vi "zad1.vi"() -> ()   [LabVIEW 2018]
uses:
  <vilib>/Instr/_visa.llb/VISA Configure Serial Port (Instr).vi
  <vilib>/measure/maspectr.llb/FFT Power Spectrum and PSD for 1 Chan.vi
  <vilib>/measure/NI_MAPro.lvlib
panel:
  out "Waveform Graph":cluster{"f0":dbl, "df":dbl, "magnitude":dbl[]}(graph)
  out "1/x":dbl
  in  "dt":dbl
  out "Waveform Graph 2":dbl[](graph)
  out "Waveform Chart 2":dbl(graph)
  out "Waveform Chart":cluster{dbl, dbl, dbl}(graph)
  in  "stop":bool
  in  "baud rate (9600)":u32=9600
  in  "VISA resource name":refnum<visa-resource-name>
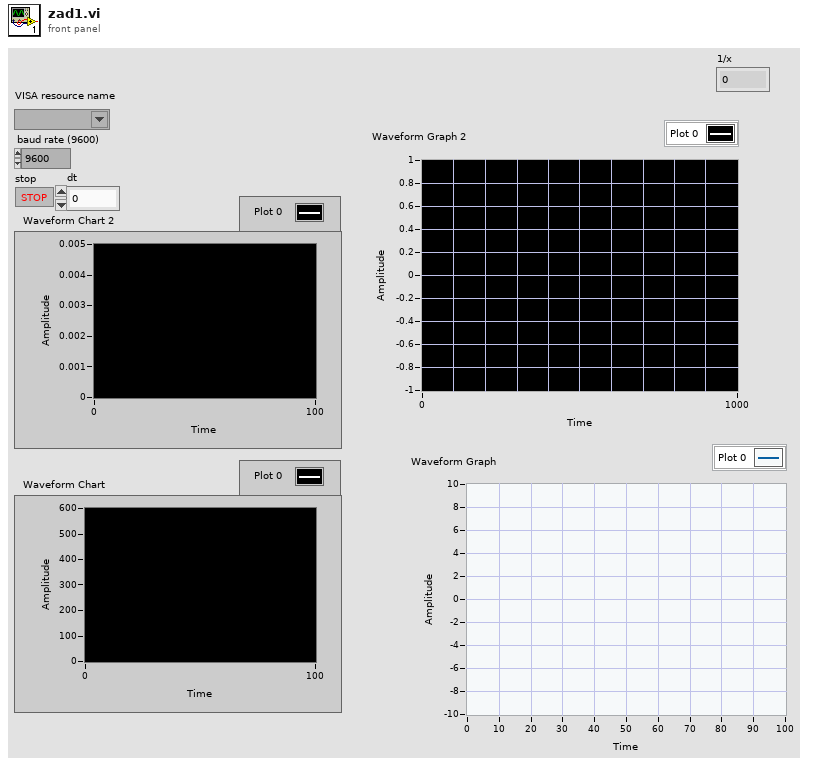
[diagram p1: front panel]
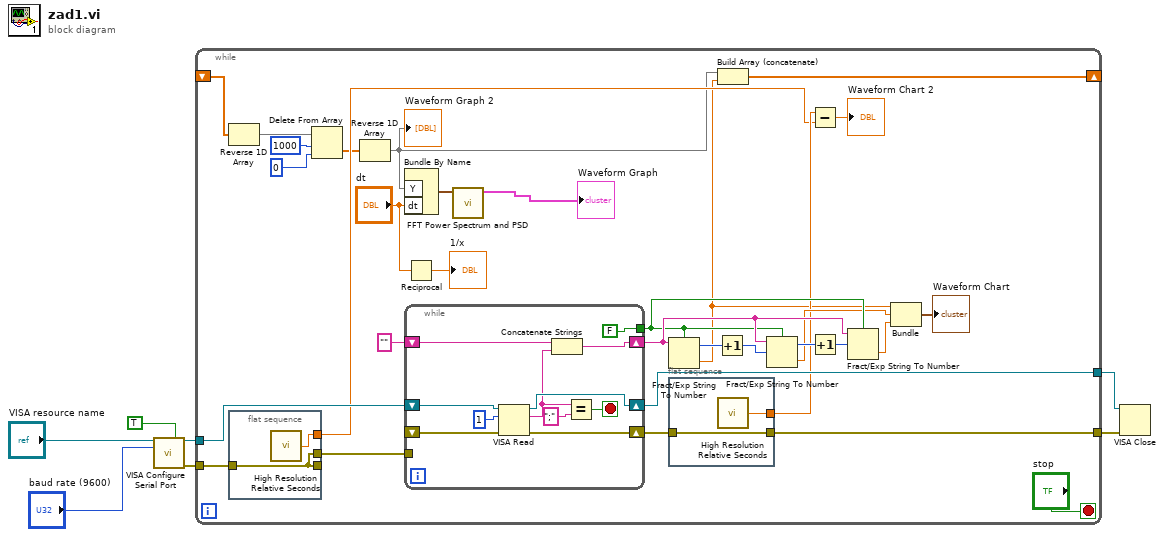
[diagram p0: block diagram]
diagram:
  n1 = call-poly "VISA Configure Serial Port"("VISA resource name"="VISA resource name", "Enable Termination\nChar (T)"=TRUE ("Enable Termination\nChar (T)"), "baud rate (9600)"="baud rate (9600)") -> ("VISA resource name out"=w2:refnum<visa-resource-name>, "error out"=w1:errorcluster)  [unwired: 11 in]
  n2 = while {
    tunnel: [w23] -> w7
    tunnel: [w39] -> w6
    tunnel: w2 -> [w27]
    tunnel: w1 -> [w26]
    shift-right: [w18] -> _
    shift-left: _ -> [w17]
    stop <- "stop" stop-if-true
    n3 = Reverse 1D Array(array=w17) -> (reversed array=w16:dbl[])
    n4 = flat-sequence {
      tunnel: [w43] -> w20
      tunnel: w26 -> [w42]
      tunnel: [w42] -> _
      tunnel: [w42] -> w25
      frame #0 {
        n5 = call <vilib>:"High Resolution Relative Seconds.vi"() -> ("relative seconds"=w43:dbl)
      }
    }
    n6 = Delete From Array(array=w16, length=1000, index=0) -> (deleted portion=w13:dbl[])  [unwired: 1 out]
    n7 = Reverse 1D Array(array=w13) -> (reversed array=w12:dbl[])
    "Waveform Graph 2" <- w12
    n8 = Bundle By Name("Y"=w12, "dt"="dt") -> (w10:waveform(dbl))  [unwired: 1 in]
    n9 = while {
      shift-right: [w53] -> w39
      shift-left: w27 -> [w54]
      shift-right: [w52] -> w24
      shift-left: _ -> [w44]
      tunnel: [FALSE ("use system decimal point (T)")] -> w31
      shift-right: [w48] -> w32
      shift-left: "" -> [w45]
      tunnel: w25 -> [_]
      stop <- w49 stop-if-true
      n10 = VISA Read(VISA resource name=w54, byte count=u32 1, error in (no error)=w44) -> (VISA resource name out=w53:refnum<visa-resource-name>, read buffer=w46:string, error out=w52:errorcluster)  [unwired: 1 out]
      n11 = Concatenate Strings(w45, w46) -> (w48:string)
      n12 = Equal?(x=w46, y=";") -> (x = y?=w49:bool)
    }
    n13 = Reciprocal(x="dt") -> (1/x=→"1/x":dbl)
    n14 = call-poly <vilib>:"FFT Power Spectrum and PSD.vi"("time signal"=w10) -> ("Power Spectrum / PSD"=→"Waveform Graph":cluster{"f0":dbl, "df":dbl, "magnitude":dbl[]})  [unwired: 7 in, 3 out]
    n15 = Fract/Exp String To Number(use system decimal point (T)=w31, string=w32) -> (offset past number=w36:i32, number=w19:dbl)  [unwired: 2 in]
    n16 = flat-sequence {
      tunnel: [w41] -> w22
      tunnel: w24 -> [w40]
      tunnel: [w40] -> w23
      frame #0 {
        n17 = call <vilib>:"High Resolution Relative Seconds.vi"() -> ("relative seconds"=w41:dbl)
      }
    }
    n18 = Increment(x=w36) -> (x+1=w35:i32)
    n19 = Build Array (concatenate)(w12, w19) -> (w18:dbl[])
    n20 = Fract/Exp String To Number(use system decimal point (T)=w31, string=w32, offset=w35) -> (offset past number=w34:i32, number=w30:dbl)  [unwired: 1 in]
    n21 = Subtract(x=w22, y=w20) -> (x-y=→"Waveform Chart 2":dbl)
    n22 = Increment(x=w34) -> (x+1=w33:i32)
    n23 = Fract/Exp String To Number(use system decimal point (T)=w31, string=w32, offset=w33) -> (number=w29:dbl)  [unwired: 1 in, 1 out]
    n24 = Bundle(w19, w30, w29) -> (→"Waveform Chart":cluster{dbl, dbl, dbl})  [unwired: 1 in]
  }
  n25 = VISA Close(VISA resource name=w6, error in (no error)=w7) -> ()  [unwired: 1 out]
